vi "Initialise.vi"(8 "error in (no error)":errorcluster, 11 "Actor in":refnum<class "Task Scheduler Actor.lvclass">) -> (0 "error out":errorcluster, 3 "Actor out":refnum<class "Task Scheduler Actor.lvclass">, 5 "Observers":cluster{"Actor":refnum<event-registration>})   [LabVIEW 2015, in "Task Scheduler Actor.lvclass"]
uses:
  Task Scheduler Actor.lvclass
  Re-use Libraries/Minimal Actor Framework/Messaging/Message/Message.lvclass
  Re-use Libraries/Utility/Utility.lvlib
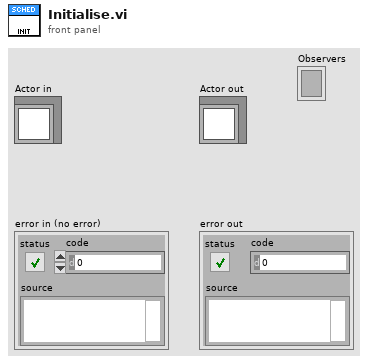
[diagram p1: front panel]
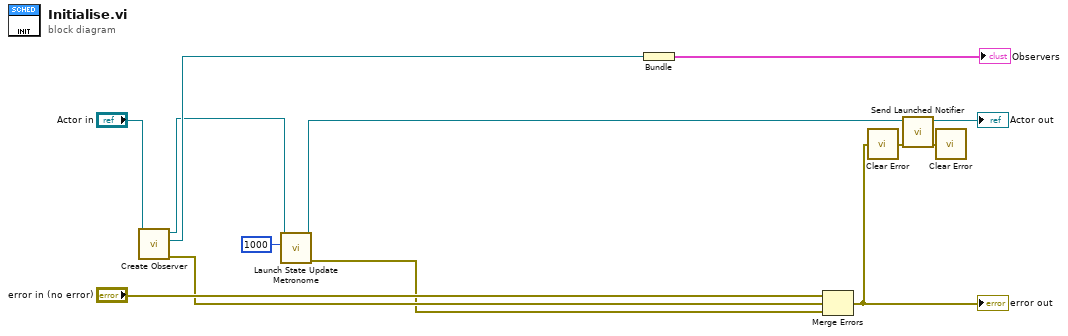
[diagram p0: block diagram]
diagram:
  n1 = call-dynamic "Create Observer.vi"("Actor in"="Actor in") -> ("error out"=w6:errorcluster, "Actor"=w7:refnum<event-registration>, "Actor out"=w4:refnum<class "Task Scheduler Actor.lvclass">)  [unwired: 8 in]
  n2 = call-dynamic "Launch State Update Metronome.vi"("Status Update Period [1000 ms]"=1000, "Actor in"=w4) -> ("error out"=w1:errorcluster, "Actor out"=w3:refnum<class "Task Scheduler Actor.lvclass">)  [unwired: 8 in]
  n3 = Bundle("Actor"=w7) -> (→"Observers":cluster{"Actor":refnum<event-registration>})  [unwired: 1 in]
  n4 = Merge Errors("error in (no error)", w6, w1) -> (w11:errorcluster)
  "error out" <- w11
  n5 = call "Clear Error.vi"("error in (no error)"=w11) -> ("error out"=w10:errorcluster)
  n6 = call-dynamic "Send Launched Notifier.vi"("error in (no error)"=w10, "Actor in"=w3) -> ("error out"=w9:errorcluster, "Actor out"=→"Actor out":refnum<class "Task Scheduler Actor.lvclass">)  [unwired: 8 in]
  n7 = call "Clear Error.vi"("error in (no error)"=w9) -> ()  [unwired: 1 out]
